vi "Fluke 6105A Set_v2.vi"(0 "VISA resource name":refnum<visa-resource-name>="6105A", 1 "Lower Range":dbl=20.0, 2 "Flicker Depth":dbl=60.0, 3 "Upper Range":dbl=50.0, 5 "Frequency":i32=50, 6 "Voltage or Current":enum16{"Voltage", "Current"}(ring), 7 "Enable Flicker?":bool, 8 "Duty Cycle":dbl=15.0, 9 "Enable Harmonics?":bool=TRUE, 10 "Reset? (T: Yes)":bool=TRUE, 11 "Harmonics":i32[](array[numeric]), 12 "Amplitudes":dbl[](array[numeric]), 13 "Flicker Frequency":dbl=40.0, 14 "Phases":dbl[](array[numeric])) -> (4 "VISA resource name out":refnum<visa-resource-name>, 15 "error out":errorcluster)   [LabVIEW 2014]
doc: "This VI is a simple example showing how to configure global settings and 2 harmonics."
uses:
  SharedVariables/TSE_Variables.vi
panel:
  in  "Shape":string(combo)="SQU"
  in  "Current Bandwidth":string(combo)="NORM"
  in  "Output Selector":u16(ring)=1 items=["L1"=1, "L2"=2, "L3"=3, "N"=4]
  in  "Sense Setting (1:4-wire)":u16(ring)=1 items=["2-wire sensing", "4-wire sensing"]
  in  "Angle Setting (0: Degrees)":string(combo)="DEG"
  in  "Line Locking (F: Off)":bool
  in  "stop":bool
  # "(c) 2004 - 2010 National Instruments.  ALL RIGHTS RESERVED."
  # "Global Settings"
  # "Voltage Harmonics Amplitude"
  # "Absolute RMS"
  # "Voltage Harmonics Amplitude"
  # "Absolute RMS"
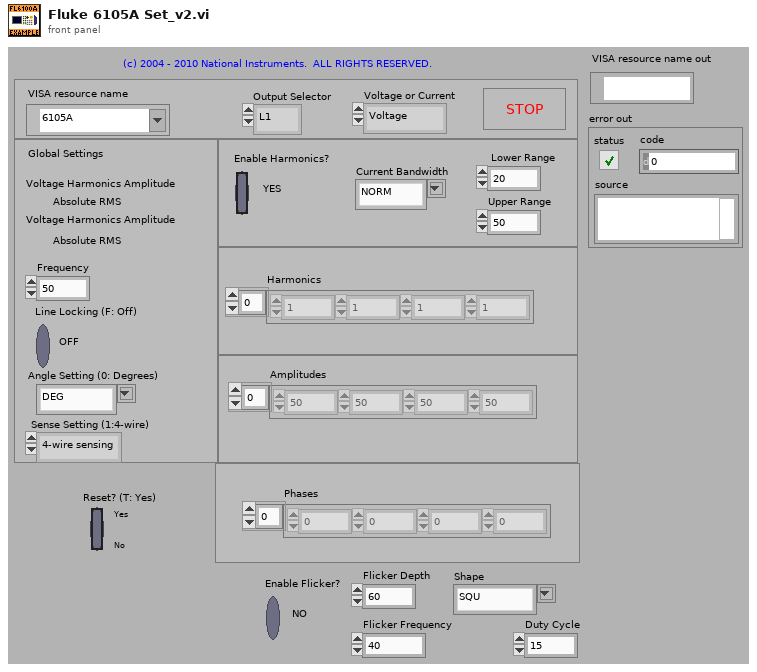
[diagram p1: front panel]
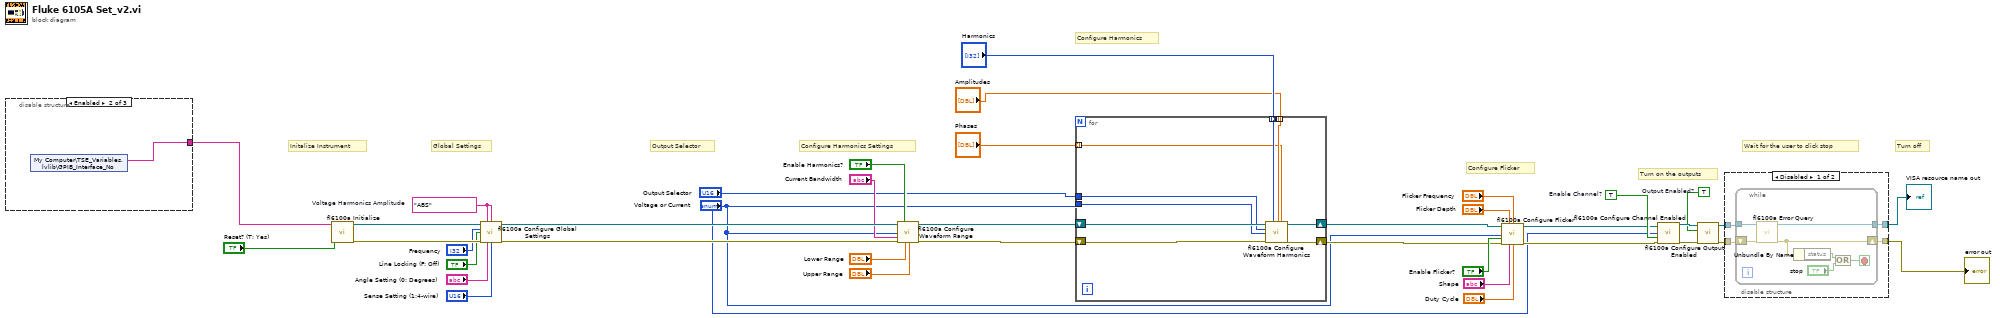
[diagram p0: block diagram]
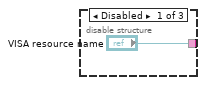
[diagram p2: hidden frame]
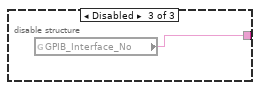
[diagram p3: hidden frame]
diagram:
  w20 = "ABS"  # Voltage Harmonics Amplitude
  w21 = TRUE  # Enable Channel?
  w22 = TRUE  # Output Enabled?
  # "Configure Flicker"
  # "Configure Harmonics"
  # "Turn off"
  # "Turn on the outputs"
  # "Wait for the user to click stop"
  # "Configure Harmonics Settings"
  # "Output Selector"
  # "Global Settings"
  # "Initalize Instrument"
  n1 = disable-structure shown="Enabled" {
    disable-tunnel: ["VISA resource name" w41 w42] -> w37
    frame Disabled {
    }
    frame Enabled {
      n2 = shared-variable "My Computer\\TSE_Variables.lvlib\\GPIB_Interface_No"() -> (w41:string)  [unwired: 1 in, 1 out]
    }
    frame Disabled {
      n3 = global read "TSE_Variables.vi" "GPIB_Interface_No"() -> (w42:string)
    }
  }
  n4 = call <instrlib>:"fl6100a Initialize.vi"("Reset? (T: Yes)"="Reset? (T: Yes)", "VISA resource name"=w37) -> ("error out"=w38:errorcluster, "VISA resource name out"=w39:refnum<visa-resource-name>)  [unwired: 8 in]
  n5 = call <instrlib>:"fl6100a Configure Global Settings.vi"("VISA resource name"=w39, "Voltage Harmonics Amplitude (0: Absolute RMS)"=w20, "Current Harmonics Amplitude (0: Absolute RMS)"=w20, "Frequency (60 Hz)"="Frequency", "Line Locking (F: Off)"="Line Locking (F: Off)", "error in (no error)"=w38, "Angle Setting (0: Degrees)"="Angle Setting (0: Degrees)", "Sense Setting (1:4-wire)"="Sense Setting (1:4-wire)") -> ("VISA resource name out"=w32:refnum<visa-resource-name>, "error out"=w31:errorcluster)  [unwired: 6 in]
  n6 = call <instrlib>:"fl6100a Configure Waveform Range.vi"("VISA resource name"=w32, "Enable Harmonics? (F:NO)"="Enable Harmonics?", "Voltage or Current (0: Voltage)"="Voltage or Current", "Current Bandwidth (1:6000 Hz)"="Current Bandwidth", "error in (no error)"=w31, "Lower Range (1)"="Lower Range", "Upper Range (2)"="Upper Range") -> ("VISA resource name out"=w30:refnum<visa-resource-name>, "error out"=w29:errorcluster)  [unwired: 7 in]
  n7 = for {
    tunnel: "Output Selector" -> [w49]
    tunnel: "Voltage or Current" -> [w48]
    shift-right: [w47] -> w3
    shift-left: w30 -> [w51]
    shift-right: [w46] -> w5
    shift-left: w29 -> [w50]
    tunnel: "Harmonics" -> [w45] mode=indexing
    tunnel: "Amplitudes" -> [w44] mode=indexing
    tunnel: "Phases" -> [w43] mode=indexing
    n8 = call <instrlib>:"fl6100a Configure Waveform Harmonics.vi"("VISA resource name"=w51, "Harmonic (1)"=w45, "Amplitude (1)"=w44, "Phase Angle (0)"=w43, "Output Selector (0:L1)"=w49, "Voltage or Current (0: Voltage)"=w48, "error in (no error)"=w50) -> ("VISA resource name out"=w47:refnum<visa-resource-name>, "error out"=w46:errorcluster)  [unwired: 7 in]
  }
  n9 = call <instrlib>:"fl6100a Configure Flicker.vi"("VISA resource name"=w3, "Flicker Depth (0 %)"="Flicker Depth", "Flicker Frequency (13.5 Hz)"="Flicker Frequency", "Voltage or Current (0: Voltage)"="Voltage or Current", "Enable Flicker? (F:NO)"="Enable Flicker?", "error in (no error)"=w5, "Flicker Shape (Sinusoidal)"="Shape", "Flicker Duty Cycle (0 %)"="Duty Cycle") -> ("VISA resource name out"=w2:refnum<visa-resource-name>, "error out"=w4:errorcluster)  [unwired: 6 in]
  n10 = call <instrlib>:"fl6100a Configure Channel Enabled.vi"("VISA resource name"=w2, "Voltage or Current (0: Voltage)"="Voltage or Current", "Enable Channel? (F:NO)"=w21, "error in (no error)"=w4) -> ("VISA resource name out"=w26:refnum<visa-resource-name>, "error out"=w23:errorcluster)  [unwired: 10 in]
  n11 = call <instrlib>:"fl6100a Configure Output Enabled.vi"("error in (no error)"=w23, "Enable Output? (F:NO)"=w22, "VISA resource name"=w26) -> ("error out"=w24:errorcluster, "VISA resource name out"=w25:refnum<visa-resource-name>)  [unwired: 7 in]
  n12 = disable-structure shown="Disabled" {
    disable-tunnel: w25 -> [w55 w64]
    disable-tunnel: w24 -> [w54 w63]
    disable-tunnel: [w53 w64] -> w17
    disable-tunnel: [w52 w63] -> w16
    frame Disabled {
      n13 = while {
        tunnel: w55 -> [w62]
        shift-right: [w60] -> w52
        shift-left: w54 -> [w61]
        tunnel: [w56] -> w53
        stop <- w57 stop-if-true
        n14 = call <instrlib>:"fl6100a Error Query.vi"("error in (no error)"=w61, "VISA resource name"=w62) -> ("error out"=w60:errorcluster, "VISA resource name out"=w56:refnum<visa-resource-name>)  [unwired: 6 in, 2 out]
        n15 = Unbundle By Name(w60) -> ("status"=w59:bool)
        n16 = Or(x=w59, y="stop") -> (x .or. y?=w57:bool)
      }
    }
    frame Enabled {
    }
  }
  "VISA resource name out" <- w17
  "error out" <- w16
